vi "from string.vi"(8 "error in":errorcluster, 9 "data":string, 10 "version":string, 11 "engine configuration in":refnum<class "engine configuration.lvclass">) -> (0 "error out":errorcluster, 3 "engine configuration out":refnum<class "engine configuration.lvclass">)   [LabVIEW 2013, in "engine configuration.lvclass"]
doc: "Takes a version and data string and unflattens the data back into an Engine Configuration object."
uses:
  engine configuration.lvclass
  Module Mappings.ctl
  <vilib>/NI/Tag Bus/table/mapping specification.ctl
  <vilib>/NI/Tag Bus/tag/Data Type.ctl
  <vilib>/NI/Tag Bus/table/mapping.ctl
  Tag Info.ctl
  <vilib>/NI/Tag Bus/tag/tag descriptor.lvclass
  <vilib>/NI/Tag Bus Module Framework/root configuration/TBM configuration.lvclass
  engine configuration.lvclass/engine configuration.ctl
  <vilib>/NI/Tag Bus/table/data table.lvlib
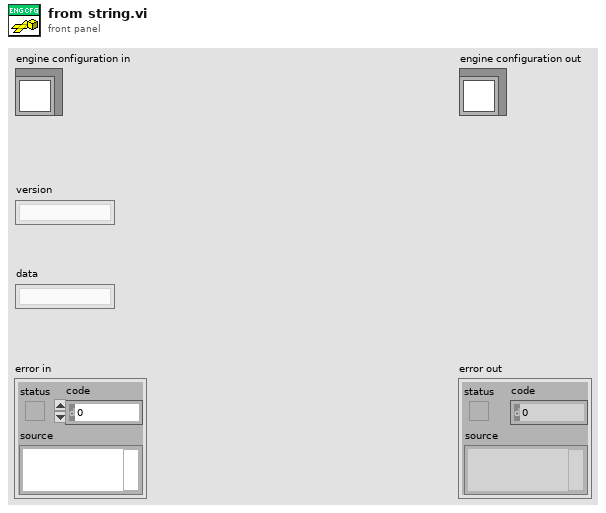
[diagram p1: front panel]
types:
  T1 = typedef "engine configuration.lvclass/Tag Info.ctl" = cluster{"Tag":refnum<class "tag descriptor.lvclass">, "Writer":string, "Readers":string[], "Owning ID":string}
  T2 = typedef "engine configuration.lvclass/Module Mappings.ctl" = cluster{"Owning ID":string, "Input Mappings":T3[], "Process Parameter Mappings":T3[], "Process Results Mappings":T3[], "Output Mappings":T3[]}
  T3 = typedef "tag bus.lvlib/data table.lvlib/mapping specification.ctl" = cluster{"data type":T4, "mappings":T5[]}
  T4 = typedef "tag bus.lvlib/tag descriptor.lvclass/Data Type.ctl" = enum16{"Double", "Single", "I64", "I32", "I16", "I8", "U64", "U32", "U16", "U8", "Boolean", "String", "Array of Double", "Array of Single", "Array of I64", "Array of I32", "Array of I16", "Array of I8", "Array of U64", "Array of U32", "Array of U16", "Array of U8", "Array of Boolean", "Array of String"}
  T5 = typedef "tag bus.lvlib/data table.lvlib/mapping.ctl" = cluster{"sink name":string, "source name":string}
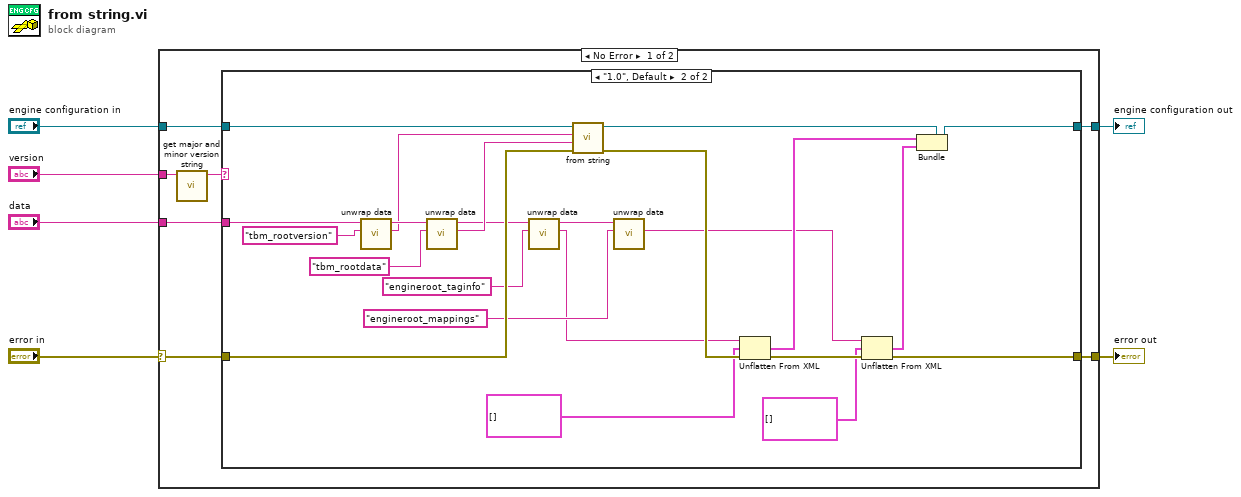
[diagram p0: block diagram]
diagram:
  n1 = case shown="No Error" "error in" {
    selector: "error in" -> [w7 w40]
    tunnel: "data" -> [w13 _]
    tunnel: "engine configuration in" -> [w12 w39]
    tunnel: [w11 w39] -> w4
    tunnel: [w10 w40] -> w3
    tunnel: "version" -> [w9 _]
    frame No Error {
      n2 = call <vilib>:"get major and minor version string.vi"("full version"=w9) -> ("major.minor version"=w8:string)  [unwired: 10 in]
      n3 = case shown="\"1.0\", Default" w8 {
        tunnel: w7 -> [w14 w38]
        tunnel: w13 -> [_ w31]
        tunnel: w12 -> [w15 w37]
        tunnel: [w15 w27] -> w11
        tunnel: [w14 w26] -> w10
        frame "False" {
        }
        frame "1.0", Default {
          n4 = call <vilib>:"unwrap data.vi"("identifier"="tbm_rootversion" ("additional identifier"), "data to unwrap"=w31) -> ("unwrapped data"=w30:string, "remaining string"=w34:string)  [unwired: 8 in]
          n5 = call <vilib>:"unwrap data.vi"("identifier"="tbm_rootdata" ("additional identifier"), "data to unwrap"=w34) -> ("unwrapped data"=w29:string, "remaining string"=w21:string)  [unwired: 8 in]
          n6 = call <vilib>:"unwrap data.vi"("identifier"="engineroot_taginfo" ("additional identifier"), "data to unwrap"=w21) -> ("unwrapped data"=w16:string, "remaining string"=w20:string)  [unwired: 8 in]
          n7 = call-parent "from string.vi"("error in"=w38, "data"=w29, "version"=w30, "configuration in"=w37) -> ("error out"=w35:errorcluster, "configuration out"=w36:refnum<class "engine configuration.lvclass">)  [unwired: 6 in]
          n8 = call <vilib>:"unwrap data.vi"("identifier"="engineroot_mappings" ("additional identifier"), "data to unwrap"=w20) -> ("unwrapped data"=w17:string)  [unwired: 8 in, 1 out]
          n9 = Unflatten From XML(xml string=w16, type=T1[] [] ("Tag List"), error in (no error)=w35) -> (value=w22:T1[], error out=w28:errorcluster)
          n10 = Unflatten From XML(xml string=w17, type=T2[] [] ("module Mappings"), error in (no error)=w28) -> (value=w24:T2[], error out=w26:errorcluster)
          n11 = Bundle(cluster=w36, w22, w24) -> (w27:refnum<class "engine configuration.lvclass">)
        }
      }
    }
    frame Error {
    }
  }
  "error out" <- w3
  "engine configuration out" <- w4
